vi "Init Queue.vi"() -> (1 "LowPriorityQueue":T1, 3 "HighPriorityQueue":T1)   [LabVIEW 2014]
uses:
  CAN Message Queue.ctl
  CAN Message.ctl
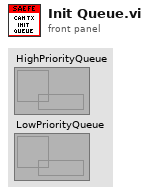
[diagram p1: front panel]
types:
  T1 = typedef "CAN Message Queue.ctl" = refnum<k33>
  T2 = typedef "CAN Message.ctl" = cluster{"identifier":u32, "extended?":bool, "type":u8, "data":cluster{"B0":u8, "B1":u8, "B2":u8, "B3":u8, "B4":u8, "B5":u8, "B6":u8, "B7":u8}}
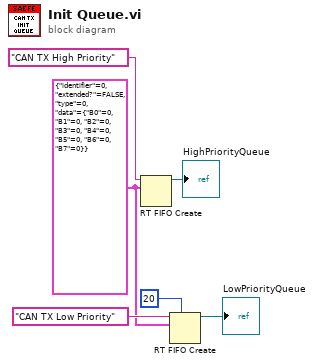
[diagram p0: block diagram]
diagram:
  w3 = T2 {"identifier"=0, "extended?"=FALSE, "type"=0, "data"={"B0"=0, "B1"=0, "B2"=0, "B3"=0, "B4"=0, "B5"=0, "B6"=0, "B7"=0}} ("CAN frame")
  n1 = RT FIFO Create(0:"CAN TX High Priority" ("name (unnamed)"), 1:w3) -> (8:→"HighPriorityQueue":refnum<k33>)  [unwired: 6 in, 2 out]
  n2 = RT FIFO Create(0:"CAN TX Low Priority" ("name (unnamed)"), 1:w3, 4:u32 20 ("size (10)")) -> (8:→"LowPriorityQueue":refnum<k33>)  [unwired: 5 in, 2 out]
